vi "sta_makeFactorsMatrix(SubVI).vi"(8 "에러 입력(에러 없음)":errorcluster, 10 "factors 입력":dbl[](array[numeric]), 11 "factors name":string[](array[string])) -> (0 "에러 출력":errorcluster, 1 "name":string[](array[string]), 2 "factors 출력":dbl[](array[numeric]), 3 "참조 번호 출력":refnum<k35>)   [LabVIEW 2018]
uses:
  PythonConfigGlobal.vi
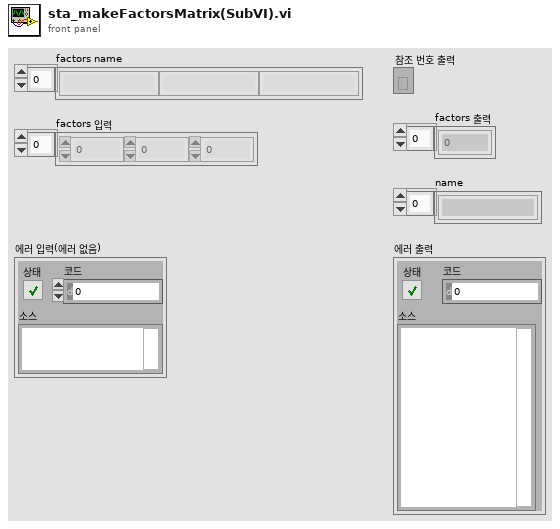
[diagram p1: front panel]
types:
  T1 = cluster{"session out":refnum<k35>, "appended path":path}
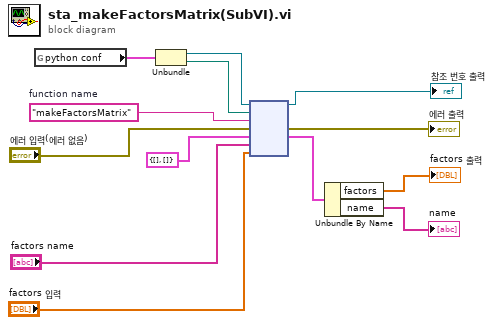
[diagram p0: block diagram]
diagram:
  w2 = "makeFactorsMatrix"  # function name
  n1 = global read "PythonConfigGlobal.vi" "python conf"() -> (w6:T1)
  n2 = Unbundle(w6) -> ("session out"=w3:refnum<k35>, "appended path"=w4:path)
  n3 = node(w3, w4, w2, "에러 입력(에러 없음)", cluster{"factors":dbl[], "name":string[]} {"factors"=[], "name"=[]}, "factors name", "factors 입력") -> (→"참조 번호 출력":refnum<k35>, →"에러 출력":errorcluster, w11:cluster{"factors":dbl[], "name":string[]})  [unwired: 2 in, 2 out]
  n4 = Unbundle By Name(w11) -> ("factors"=→"factors 출력":dbl[], "name"=→"name":string[])
